vi "MV3D RGBD Get SDK Version.vi"(11 "pstVersion":T1) -> (2 "function return":i32, 3 "pstVersion out":T1)   [LabVIEW 2015, in "Mv3dRgbd.lvlib"]
doc: "MV3D_RGBD_API MV3D_RGBD_STATUS MV3D_RGBD_GetSDKVersion(MV3D_RGBD_VERSION_INFO* pstVersion);"
uses:
  <userlib>/Mv3dRgbd/Mv3dRgbd.lvlib
  <userlib>/Mv3dRgbd/Mv3dRgbd.dll
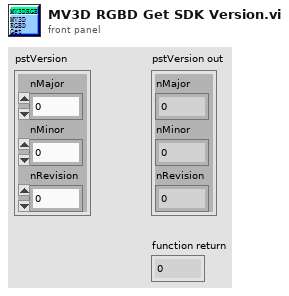
[diagram p1: front panel]
types:
  T1 = cluster{"nMajor":u32, "nMinor":u32, "nRevision":u32}
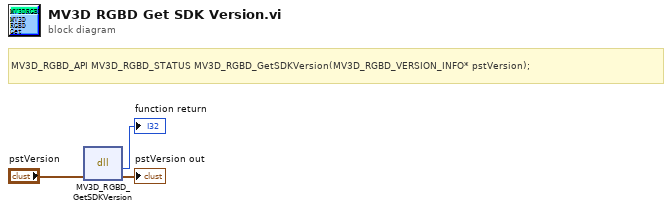
[diagram p0: block diagram]
diagram:
  # "MV3D_RGBD_API MV3D_RGBD_STATUS MV3D_RGBD_GetSDKVersion(MV3D_RGBD_VERSION_INFO* pstVersion);"
  n1 = dll-call lib="C:/Program Files (x86)/National Instruments/LabVIEW 2015/user.lib/Mv3dRgbd/Mv3dRgbd.*" fn="MV3D_RGBD_GetSDKVersion"("pstVersion"="pstVersion") -> (→"function return":i32, "pstVersion"=→"pstVersion out":T1)  [unwired: 3 in, 2 out]
